vi "Valid Attributes Metadata.vi"(10 "Attributes Metadata":refnum<class "Attributes Metadata.lvclass">) -> (2 "Valid Attributes Metadata":bool)   [LabVIEW 2020, in "jettl.lvlib"]
uses:
  jettl.lvlib
  Attributes Metadata/Attributes Metadata.lvclass
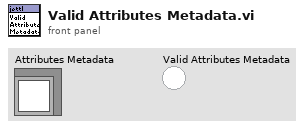
[diagram p1: front panel]
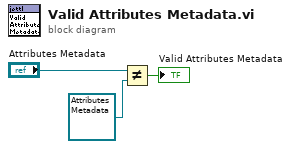
[diagram p0: block diagram]
diagram:
  n1 = Not Equal?(x="Attributes Metadata", y=refnum<class "Attributes Metadata.lvclass"> refnum) -> (x != y?=→"Valid Attributes Metadata":bool)
